vi "test Get Owning Custom Device.vi"(8 "error in":errorcluster, 11 "TestCase in":refnum<class "Scripting.lvclass">) -> (0 "error out":errorcluster, 3 "TestCase out":refnum<class "Scripting.lvclass">)   [LabVIEW 2020, in "Scripting.lvclass"]
uses:
  Scripting.lvclass
  Scripting.lvclass/Scripting.ctl
  <vilib>/addons/_JKI Toolkits/VI Tester/TestCase.llb/TestCase.lvclass
  Scripting/Ballard ARINC 429 Scripting.lvlib
  C:/Program Files (x86)/National Instruments/LabVIEW 2020/vi.lib/addons/_JKI Toolkits/VI Tester/TestCase.llb/TestCase.lvclass
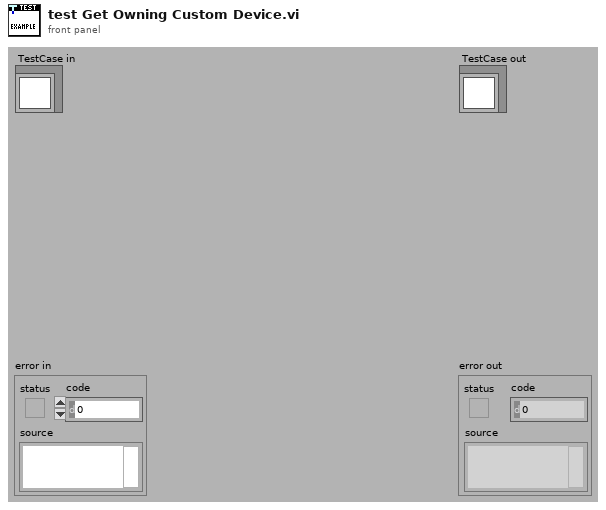
[diagram p1: front panel]
types:
  T1 = typedef "Custom Device API.lvlib/Custom Device Item Ref.ctl" = u64
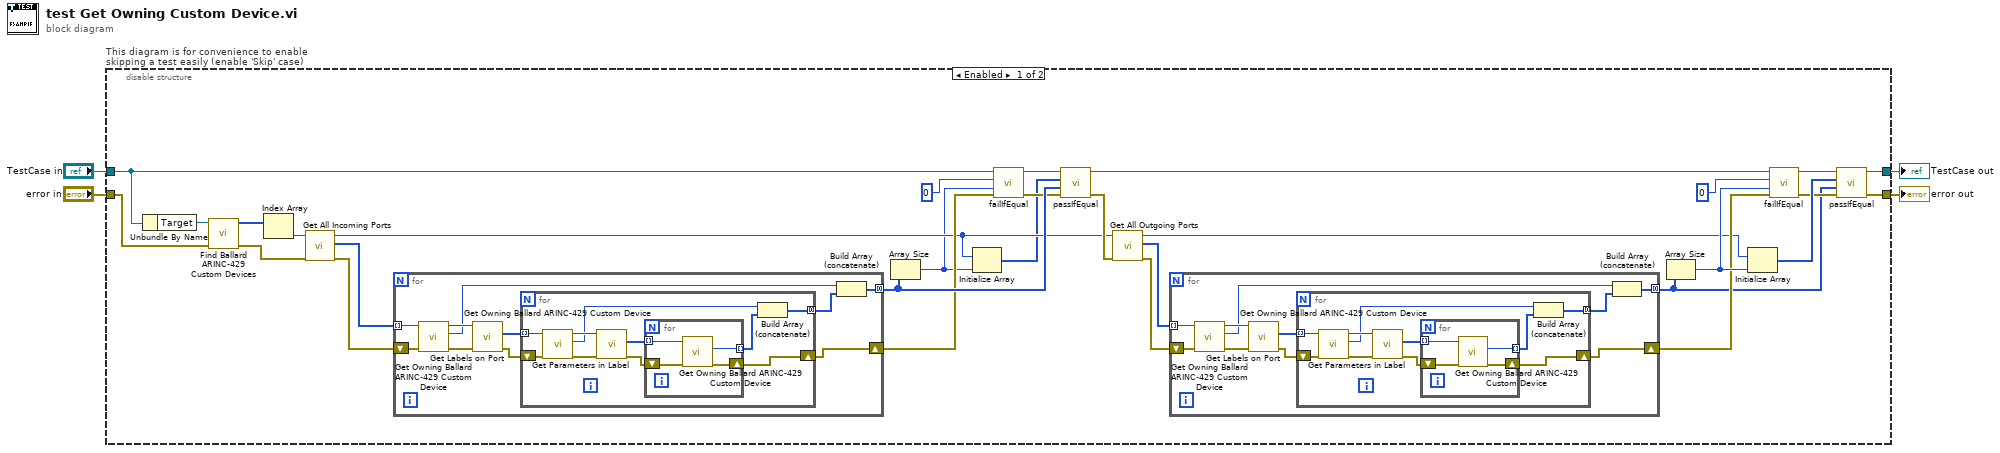
[diagram p0: block diagram]
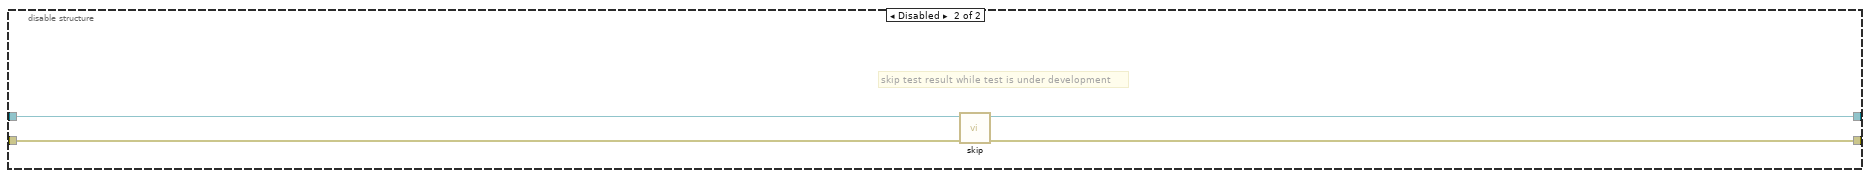
[diagram p2: hidden frame]
diagram:
  n1 = disable-structure "This diagram is for convenience to enable skipping a test easily (enable 'Skip' case)" shown="Enabled" {
    disable-tunnel: "TestCase in" -> [w23 w86]
    disable-tunnel: [w5 w84] -> w1
    disable-tunnel: [w6 w85] -> w3
    disable-tunnel: "error in" -> [w28 w83]
    frame Enabled {
      n2 = Unbundle By Name(w23) -> ("Target"=w34:refnum<k24>)
      n3 = call "Find Ballard ARINC-429 Custom Devices.vi"("error in"=w28, "target"=w34) -> ("error out"=w31:errorcluster, "Ballard ARINC-429 custom devices"=w32:u64[])  [unwired: 8 in]
      n4 = Index Array(array=w32) -> (element=w33:u64)  [unwired: 1 in]
      n5 = call "Get All Incoming Ports.vi"("error in"=w31, "Ballard ARINC 429 ref"=w33) -> ("error out"=w30:errorcluster, "Port refs"=w29:T1[], "Ballard ARINC 429 ref out"=w20:T1)  [unwired: 7 in]
      n6 = for {
        tunnel: w29 -> [w68] mode=indexing
        shift-right: [w62] -> w22
        shift-left: w30 -> [w67]
        tunnel: [w59] -> w26 mode=concatenating
        n7 = call "Get Owning Ballard ARINC-429 Custom Device.vi"("error in"=w67, "item ref in"=w68) -> ("error out"=w65:errorcluster, "owning Ballard ARINC-429 custom device"=w60:T1, "item ref out"=w66:T1)  [unwired: 7 in]
        n8 = call "Get Labels on Port.vi"("error in"=w65, "port ref"=w66) -> ("error out"=w63:errorcluster, "label references"=w64:T1[])  [unwired: 6 in, 2 out]
        n9 = for {
          tunnel: w64 -> [w78] mode=indexing
          shift-right: [w74] -> w62
          shift-left: w63 -> [w76]
          tunnel: [w69] -> w61 mode=concatenating
          n10 = call "Get Owning Ballard ARINC-429 Custom Device.vi"("error in"=w76, "item ref in"=w78) -> ("error out"=w75:errorcluster, "owning Ballard ARINC-429 custom device"=w71:T1, "item ref out"=w77:T1)  [unwired: 7 in]
          n11 = call "Get Parameters in Label.vi"("error in"=w75, "label ref"=w77) -> ("error out"=w72:errorcluster, "parameter references"=w73:T1[])  [unwired: 6 in, 2 out]
          n12 = for {
            tunnel: w73 -> [w82] mode=indexing
            tunnel: [w81] -> w70 mode=indexing
            shift-right: [w79] -> w74
            shift-left: w72 -> [w80]
            n13 = call "Get Owning Ballard ARINC-429 Custom Device.vi"("error in"=w80, "item ref in"=w82) -> ("error out"=w79:errorcluster, "owning Ballard ARINC-429 custom device"=w81:T1)  [unwired: 7 in, 1 out]
          }
          n14 = Build Array (concatenate)(w71, w70) -> (w69:T1[])
        }
        n15 = Build Array (concatenate)(w60, w61) -> (w59:T1[])
      }
      n16 = Array Size(array=w26) -> (size(s)=w19:i32)
      n17 = Initialize Array(w20, w19) -> (w18:T1[])
      n18 = call-dynamic "failIfEqual.vi"("error in (no error)"=w22, "y"=w19, "x"=0 ("size(s)"), "TestCase in"=w23) -> ("error out"=w21:errorcluster, "TestCase out"=w24:refnum<class "Scripting.lvclass">)  [unwired: 6 in]
      n19 = call-dynamic "passIfEqual.vi"("error in (no error)"=w21, "y"=w26, "x"=w18, "TestCase in"=w24) -> ("error out"=w27:errorcluster, "TestCase out"=w8:refnum<class "Scripting.lvclass">)  [unwired: 6 in]
      n20 = call "Get All Outgoing Ports.vi"("error in"=w27, "Ballard ARINC 429 ref"=w20) -> ("error out"=w10:errorcluster, "Port refs"=w9:T1[], "Ballard ARINC 429 ref out"=w7:T1)  [unwired: 7 in]
      n21 = for {
        tunnel: w9 -> [w44] mode=indexing
        shift-right: [w38] -> w14
        shift-left: w10 -> [w43]
        tunnel: [w35] -> w11 mode=concatenating
        n22 = call "Get Owning Ballard ARINC-429 Custom Device.vi"("error in"=w43, "item ref in"=w44) -> ("error out"=w41:errorcluster, "owning Ballard ARINC-429 custom device"=w36:T1, "item ref out"=w42:T1)  [unwired: 7 in]
        n23 = call "Get Labels on Port.vi"("error in"=w41, "port ref"=w42) -> ("error out"=w39:errorcluster, "label references"=w40:T1[])  [unwired: 6 in, 2 out]
        n24 = for {
          tunnel: w40 -> [w54] mode=indexing
          shift-right: [w50] -> w38
          shift-left: w39 -> [w52]
          tunnel: [w45] -> w37 mode=concatenating
          n25 = call "Get Owning Ballard ARINC-429 Custom Device.vi"("error in"=w52, "item ref in"=w54) -> ("error out"=w51:errorcluster, "owning Ballard ARINC-429 custom device"=w47:T1, "item ref out"=w53:T1)  [unwired: 7 in]
          n26 = call "Get Parameters in Label.vi"("error in"=w51, "label ref"=w53) -> ("error out"=w48:errorcluster, "parameter references"=w49:T1[])  [unwired: 6 in, 2 out]
          n27 = for {
            tunnel: w49 -> [w58] mode=indexing
            tunnel: [w57] -> w46 mode=indexing
            shift-right: [w55] -> w50
            shift-left: w48 -> [w56]
            n28 = call "Get Owning Ballard ARINC-429 Custom Device.vi"("error in"=w56, "item ref in"=w58) -> ("error out"=w55:errorcluster, "owning Ballard ARINC-429 custom device"=w57:T1)  [unwired: 7 in, 1 out]
          }
          n29 = Build Array (concatenate)(w47, w46) -> (w45:T1[])
        }
        n30 = Build Array (concatenate)(w36, w37) -> (w35:T1[])
      }
      n31 = Array Size(array=w11) -> (size(s)=w16:i32)
      n32 = Initialize Array(w7, w16) -> (w17:T1[])
      n33 = call-dynamic "failIfEqual.vi"("error in (no error)"=w14, "y"=w16, "x"=0 ("size(s)"), "TestCase in"=w8) -> ("error out"=w15:errorcluster, "TestCase out"=w13:refnum<class "Scripting.lvclass">)  [unwired: 6 in]
      n34 = call-dynamic "passIfEqual.vi"("error in (no error)"=w15, "y"=w11, "x"=w17, "TestCase in"=w13) -> ("error out"=w6:errorcluster, "TestCase out"=w5:refnum<class "Scripting.lvclass">)  [unwired: 6 in]
    }
    frame Disabled {
      # "skip test result while test is under development"
      n35 = call <vilib>:"skip.vi"("error in (no error)"=w83, "TestCase in"=w86) -> ("error out"=w85:errorcluster, "TestCase out"=w84:refnum<class "Scripting.lvclass">)  [unwired: 8 in]
    }
  }
  "error out" <- w3
  "TestCase out" <- w1
